vi "Presure_honeywell.vi"() -> (3 "Presure(kp)":dbl)   [LabVIEW 2014]
panel:
  out "number":dbl
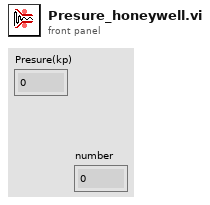
[diagram p1: front panel]
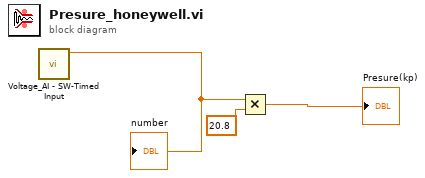
[diagram p0: block diagram]
diagram:
  n1 = call "Voltage_AI - SW-Timed Input.vi"() -> ("Waveform Chart"=w2:dbl)  [unwired: 11 in]
  "number" <- w2
  n2 = Multiply(x=w2, y=20.8) -> (x*y=→"Presure(kp)":dbl)
